vi "Generic_TR.vi"() -> ()   [LabVIEW 2018]
panel:
  out "Graph":u16[](graph)
  in  "stop":bool
  # "Connect proper signal to channel A before starting acquisition\n(e.g. 1Vpp 1kHz sine wave)"
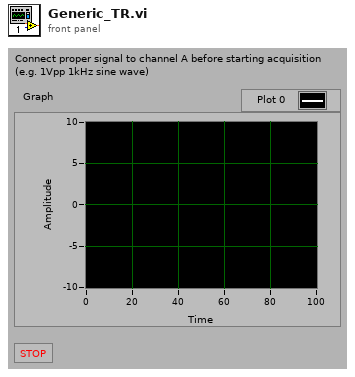
[diagram p1: front panel]
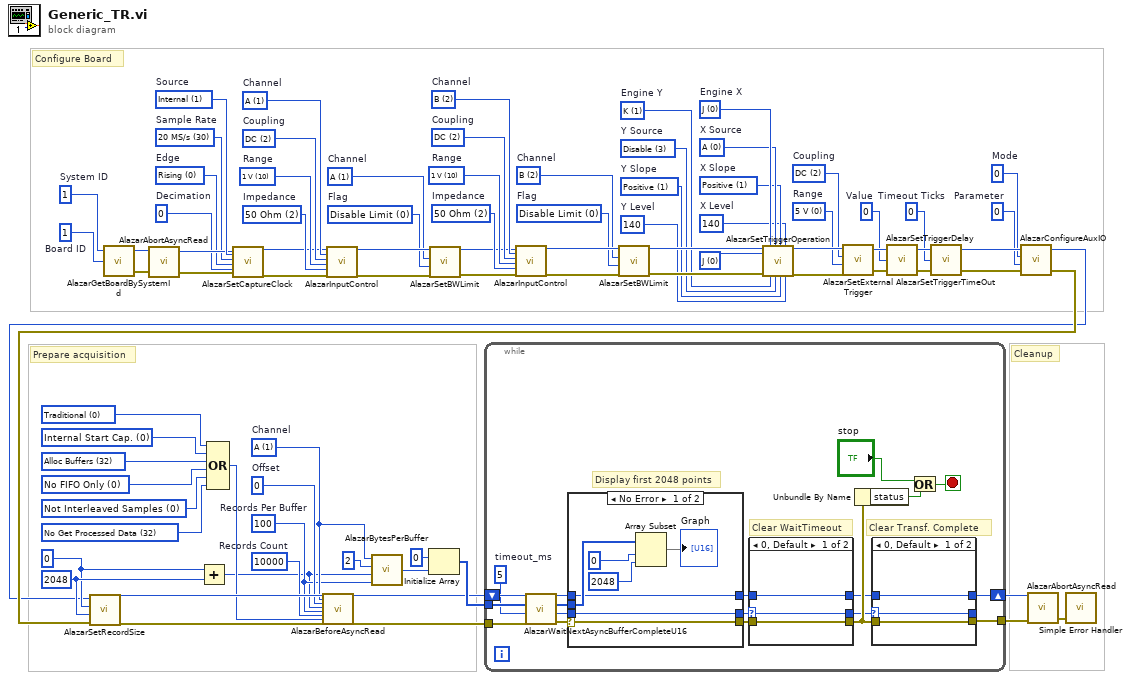
[diagram p0: block diagram]
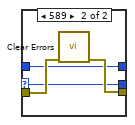
[diagram p2: hidden frame]
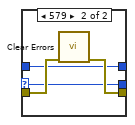
[diagram p3: hidden frame]
diagram:
  w17 = u32 10000  # Records Count
  w14 = u32 100  # Records Per Buffer
  w18 = u32 0  # Offset
  w16 = u32 1 items=["A"=1, "B"=2, "A + B"=3, "C"=4, "A + C"=5, "A + B"=6, "D"=8, "A + D"=9, "B + D"=10, "C + D"=12, "A + B + C + D"=15]  # Channel
  w23 = u32 2048 ("Post-trigger Samples")
  w22 = u32 0 ("Pre-trigger Samples")
  w27 = u32 32 items=["No Get Processed Data"=32, "Get Processed Data"=8192]
  w26 = u32 0 items=["Not Interleaved Samples"=0, "Interleave Samples"=4096]
  w24 = u32 0 items=["No FIFO Only"=0, "FIFO Only"=2048]
  w25 = u32 32 items=["Alloc Buffers"=32]
  w2 = u32 0 items=["Internal Start Cap.", "External Start Cap."]
  w1 = u32 0 items=["Traditional"=0, "NPT"=512, "Continuous"=256, "Triggered Streaming"=1024]
  w57 = u32 0 items=["Disable Limit", "Enable Limit"]  # Flag
  w56 = u32 2 items=["A"=1, "B"=2, "C"=4, "D"=8]  # Channel
  w60 = u32 2 items=["1 MOhm"=1, "50 Ohm"=2]  # Impedance
  w54 = u32 10 items=["20 mV"=1, "40 mV"=2, "50 mV"=3, "80 mV"=4, "100 mV"=5, "200 mV"=6, "400 mV"=7, "500 mV"=8, "800 mV"=9, "1 V"=10, "1.25 V"=33, "2 V"=11, "4 V"=12, "5 V"=13, "8 V"=14, "10 V"=15, "20 V"=16]  # Range
  w61 = u32 2 items=["AC"=1, "DC"=2]  # Coupling
  w62 = u8 2 items=["A"=1, "B"=2, "C"=4, "D"=8]  # Channel
  w30 = u32 0  # Parameter
  w29 = u32 0  # Mode
  w28 = u32 0  # Timeout Ticks
  w35 = u32 0  # Value
  w39 = u32 0 items=["5 V", "1 V", "TTL"]  # Range
  w38 = u32 2 items=["AC"=1, "DC"=2]  # Coupling
  w42 = u32 140  # Y Level
  w43 = u32 1 items=["Positive"=1, "Negative"=2]  # Y Slope
  w44 = u32 3 items=["A", "B", "External", "Disable", "C", "D"]  # Y Source
  w46 = u32 140  # X Level
  w47 = u32 1 items=["Positive"=1, "Negative"=2]  # X Slope
  w48 = u32 0 items=["A", "B", "External", "Disable", "C", "D"]  # X Source
  w45 = u32 1 items=["J", "K"]  # Engine Y
  w49 = u32 0 items=["J", "K"]  # Engine X
  w50 = u32 0 items=["J", "K", "J OR K", "J AND K", "J XOR K", "J AND NOT K", "NOT J AND K"] ("Op.")
  w64 = u32 0 items=["Disable Limit", "Enable Limit"]  # Flag
  w63 = u32 1 items=["A"=1, "B"=2, "C"=4, "D"=8]  # Channel
  w69 = u32 2 items=["1 MOhm"=1, "50 Ohm"=2]  # Impedance
  w70 = u32 10 items=["20 mV"=1, "40 mV"=2, "50 mV"=3, "80 mV"=4, "100 mV"=5, "200 mV"=6, "400 mV"=7, "500 mV"=8, "800 mV"=9, "1 V"=10, "1.25 V"=33, "2 V"=11, "4 V"=12, "5 V"=13, "8 V"=14, "10 V"=15, "20 V"=16]  # Range
  w71 = u32 2 items=["AC"=1, "DC"=2]  # Coupling
  w72 = u8 1 items=["A"=1, "B"=2, "C"=4, "D"=8]  # Channel
  w74 = u32 0  # Decimation
  w75 = u32 0 items=["Rising", "Falling"]  # Edge
  w76 = u32 30 items=["1 kS/s"=1, "2 kS/s"=2, "5 kS/s"=4, "10 kS/s"=8, "20 kS/s"=10, "50 kS/s"=12, "100 kS/s"=14, "200 kS/s"=16, "500 kS/s"=18, "1 MS/s"=20, "2 MS/s"=24, "5 MS/s"=26, "10 MS/s"=28, "20 MS/s"=30, "25 MS/s"=33, "50 MS/s"=34, "100 MS/s"=36, "125 MS/s"=37, "160 MS/s"=38, "180 MS/s"=39, "250 MS/s"=43, "500 MS/s"=48, "800 MS/s"=50, "1000 MS/s"=53, "1200 MS/s"=55, "1500 MS/s"=58, "1800 MS/s"=61, "USER_DEF"=0]  # Sample Rate
  w78 = u32 1 items=["Internal"=1, "Fast External"=2, "Medium External"=3, "Slow External"=4, "External AC"=5, "External DC"=6, "External 10MHz"=7]  # Source
  w82 = u32 1  # Board ID
  w81 = u32 1  # System ID
  # "Cleanup"
  # "Prepare acquisition"
  # "Configure Board"
  n1 = call "AlazarGetBoardBySystemId.vi"("Board ID"=w82, "System ID"=w81) -> ("error out"=w79:errorcluster, "Handle"=w80:u32)  [unwired: 1 in, 1 out]
  n2 = call "AlazarAbortAsyncRead.vi"("Handle"=w80, "error in (no error)"=w79) -> ("Handle"=w77:u32, "error out"=w73:errorcluster)  [unwired: 1 out]
  n3 = Add(x=w22, y=w23) -> (x+y=w3:u32)
  n4 = Compound Arithmetic op=OR(w1, w2, w25, w24, w26, w27) -> (w19:u32)
  n5 = call "AlazarSetCaptureClock.vi"("Handle"=w77, "Source"=w78, "Sample Rate"=w76, "Edge"=w75, "Decimation"=w74, "error in (no error)"=w73) -> ("Handle"=w68:u32, "error out"=w67:errorcluster)  [unwired: 11 in, 1 out]
  n6 = call "AlazarInputControl.vi"("Handle"=w68, "Channel"=w72, "Coupling"=w71, "Range"=w70, "Impedance"=w69, "error in (no error)"=w67) -> ("Handle"=w66:u32, "error out"=w65:errorcluster)  [unwired: 11 in, 1 out]
  n7 = call "AlazarBytesPerBuffer.vi"("Records Per Buffer"=w14, "Samples Per Record"=w3, "Bytes Per Sample"=u32 2, "Channel Mask"=w16) -> ("Bytes Per Buffer"=w13:u32)
  n8 = Initialize Array(u16 0, w13) -> (w11:u16[])
  n9 = call "AlazarSetBWLimit.vi"("error in (no error)"=w65, "Flag"=w64, "Channel"=w63, "Handle"=w66) -> ("error out"=w55:errorcluster, "Handle"=w53:u32)  [unwired: 1 out]
  n10 = call "AlazarInputControl.vi"("Handle"=w53, "Channel"=w62, "Coupling"=w61, "Range"=w54, "Impedance"=w60, "error in (no error)"=w55) -> ("Handle"=w59:u32, "error out"=w58:errorcluster)  [unwired: 11 in, 1 out]
  n11 = call "AlazarSetBWLimit.vi"("error in (no error)"=w58, "Flag"=w57, "Channel"=w56, "Handle"=w59) -> ("error out"=w51:errorcluster, "Handle"=w52:u32)  [unwired: 1 out]
  n12 = call "AlazarSetTriggerOperation.vi"("Handle"=w52, "Trigger Operation"=w50, "error in (no error)"=w51, "Trigger Engine 1"=w49, "Trigger Engine 2"=w45, "Source 1"=w48, "Source 2"=w44, "Slope 1"=w47, "Slope 2"=w43, "Level 1"=w46, "Level 2"=w42) -> ("Handle"=w41:u32, "error out"=w40:errorcluster)  [unwired: 6 in, 1 out]
  n13 = call "AlazarSetExternalTrigger.vi"("error in (no error)"=w40, "Range ID"=w39, "Coupling ID"=w38, "Handle"=w41) -> ("error out"=w36:errorcluster, "Handle"=w37:u32)  [unwired: 1 out]
  n14 = call "AlazarSetTriggerDelay.vi"("error in (no error)"=w36, "Delay"=w35, "Handle"=w37) -> ("error out"=w33:errorcluster, "Handle"=w34:u32)  [unwired: 1 out]
  n15 = call "AlazarSetTriggerTimeOut.vi"("error in (no error)"=w33, "Timeout Ticks"=w28, "Handle"=w34) -> ("error out"=w31:errorcluster, "Handle"=w32:u32)  [unwired: 1 out]
  n16 = call "AlazarConfigureAuxIO.vi"("error in (no error)"=w31, "Parameter"=w30, "Mode"=w29, "Handle"=w32) -> ("error out"=w5:errorcluster, "Handle"=w4:u32)  [unwired: 1 out]
  n17 = call "AlazarSetRecordSize.vi"("error in (no error)"=w5, "Post-trigger Samples"=w23, "Pre-trigger Samples"=w22, "Handle"=w4) -> ("error out"=w20:errorcluster, "Handle"=w21:u32)  [unwired: 1 out]
  n18 = call "AlazarBeforeAsyncRead.vi"("Handle"=w21, "Channel Select"=w16, "Transfer Offset"=w18, "Transfer Length"=w3, "Records Per Buffer"=w14, "Records Per Acquisition"=w17, "Flags"=w19, "error in (no error)"=w20) -> ("Handle"=w10:u32, "error out"=w9:errorcluster)  [unwired: 17 in, 1 out]
  n19 = while {
    tunnel: w11 -> [w101]
    tunnel: w9 -> [w98]
    tunnel: [w83] -> w6
    shift-right: [w84] -> w7
    shift-left: w10 -> [w100]
    stop <- w87 stop-if-true
    w99 = u32 5  # timeout_ms
    # "Clear Transf. Complete"
    # "Clear WaitTimeout"
    # "Display first 2048 points"
    n20 = call "AlazarWaitNextAsyncBufferCompleteU16.vi"("error in (no error)"=w98, "Timeout (ms)"=w99, "Buffer"=w101, "Handle"=w100) -> ("error out"=w97:errorcluster, "Return Code"=w96:u32, "Buffer"=w91:u16[], "Handle"=w93:u32)
    n21 = case shown="No Error" w97 {
      selector: w97 -> [w116 w124]
      tunnel: w96 -> [w118 w125]
      tunnel: [w118 w125] -> w95
      tunnel: [w116 w124] -> w94
      tunnel: [w117 w123] -> w92
      tunnel: w93 -> [w117 w123]
      tunnel: w91 -> [w121 _]
      frame No Error {
        n22 = Array Subset(array=w121, index=0, length=2048) -> (→"Graph":u16[])
      }
      frame Error {
      }
    }
    n23 = case shown="0, Default" w95 {
      selector: w95 -> [w110 w112]
      tunnel: w94 -> [w109 w115]
      tunnel: [w109 w114] -> w90
      tunnel: [w111 w113] -> w89
      tunnel: w92 -> [w111 w113]
      tunnel: [w110 w112] -> w88
      frame 0, Default {
      }
      frame 579 {
        n24 = call <vilib>:"Clear Errors.vi"("error in (no error)"=w115) -> ("error out"=w114:errorcluster)  [unwired: 5 in, 1 out]
      }
    }
    n25 = Unbundle By Name(w90) -> ("status"=w85:bool)
    n26 = case shown="0, Default" w88 {
      selector: w88 -> [w103 w105]
      tunnel: w90 -> [w102 w108]
      tunnel: [w102 w107] -> w83
      tunnel: [w104 w106] -> w84
      tunnel: w89 -> [w104 w106]
      tunnel: [w103 w105] -> _
      frame 0, Default {
      }
      frame 589 {
        n27 = call <vilib>:"Clear Errors.vi"("error in (no error)"=w108) -> ("error out"=w107:errorcluster)  [unwired: 5 in, 1 out]
      }
    }
    n28 = Or(x="stop", y=w85) -> (x .or. y?=w87:bool)
  }
  n29 = call "AlazarAbortAsyncRead.vi"("Handle"=w7, "error in (no error)"=w6) -> ("error out"=w8:errorcluster)  [unwired: 2 out]
  n30 = call <vilib>:"Simple Error Handler.vi"("error in (no error)"=w8) -> ()  [unwired: 4 in, 5 out]
